vi "joystick benchmark test.vi"() -> ()   [LabVIEW 2015]
uses:
  <vilib>/Utility/inputDevices.llb/closeJoystick.vi
panel:
  out "joystick info":T1(array[cluster])
  out "device ID":refnum<k1>
  out "Numeric":u32
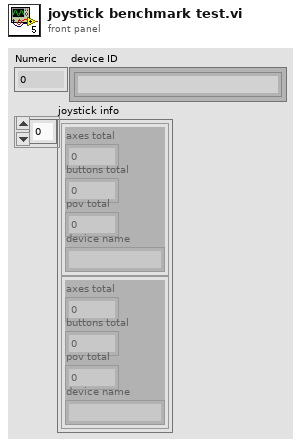
[diagram p1: front panel]
types:
  T1 = cluster{"axes total":u32, "buttons total":u32, "pov total":u32, "device name":string}[]
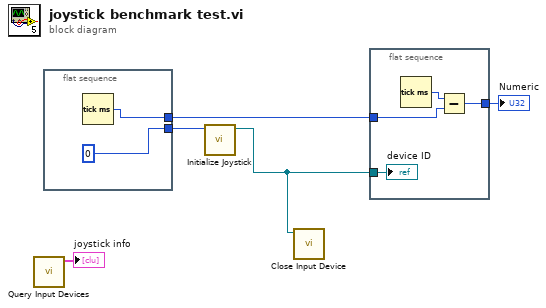
[diagram p0: block diagram]
diagram:
  n1 = call <vilib>:"Query Input Devices.vi"() -> ("joystick info"=→"joystick info":T1)  [unwired: 8 in, 3 out]
  n2 = flat-sequence {
    tunnel: [0 ("device index")] -> w5
    tunnel: [w6] -> w4
    frame #0 {
      n3 = Tick Count (ms)() -> (millisecond timer value=w6:u32)
    }
  }
  n4 = call <vilib>:"Initialize Joystick.vi"("device index"=w5) -> ("device ID"=w2:refnum<k1>)  [unwired: 1 in, 9 out]
  n5 = call-poly <vilib>:"Close Input Device.vi"("device ID"=w2) -> ()  [unwired: 9 in, 1 out]
  n6 = flat-sequence {
    tunnel: w2 -> [w8]
    tunnel: w4 -> [w10]
    tunnel: [w9] -> w3
    frame #0 {
      n7 = Tick Count (ms)() -> (millisecond timer value=w11:u32)
      n8 = Subtract(x=w11, y=w10) -> (x-y=w9:u32)
      "device ID" <- w8
    }
  }
  "Numeric" <- w3
